vi "validate inputs.vi"(9 "output in":T3, 10 "process in":T1, 11 "input in":T2) -> (1 "output out":T3, 2 "process out":T1, 3 "input out":T2)   [LabVIEW 2013]
uses:
  Controls/output script control.ctl
  Controls/input script control.ctl
  Controls/processing script control.ctl
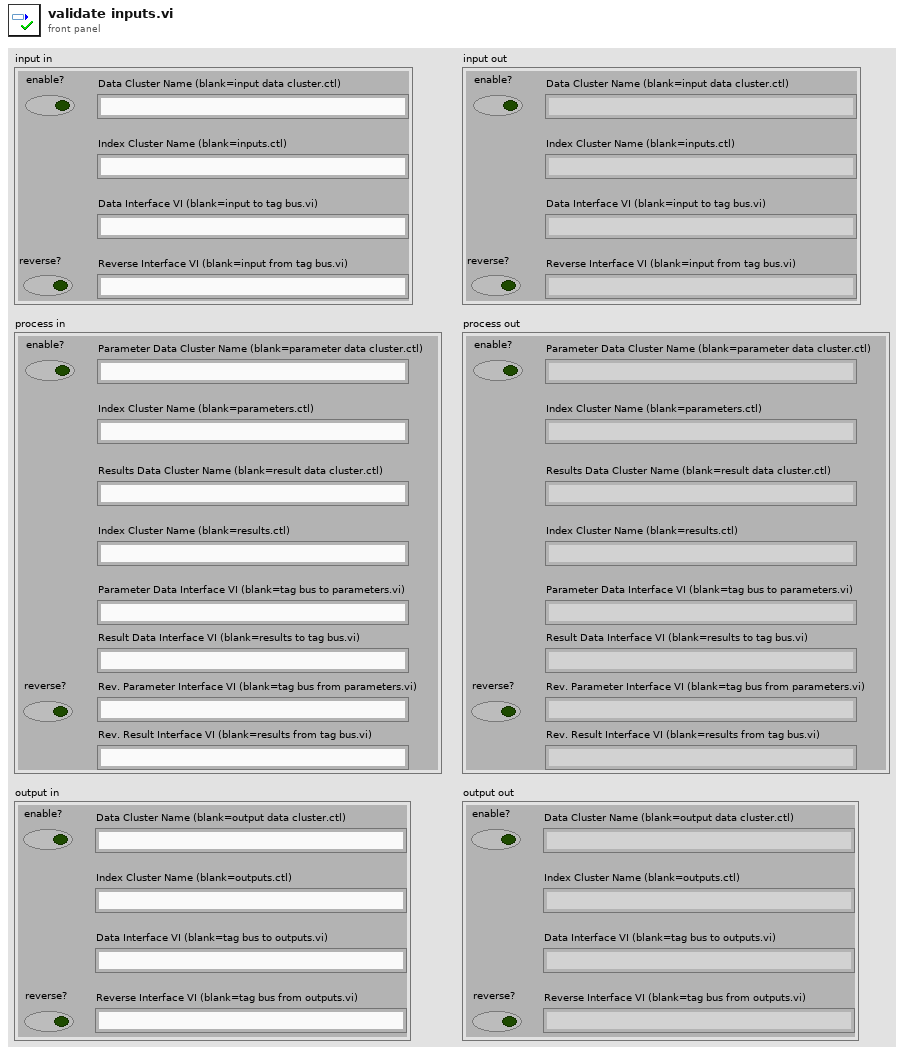
[diagram p1: front panel]
types:
  T1 = typedef "processing script control.ctl" = cluster{"enable?":bool, "Parameter Data Cluster Name (blank=parameter data cluster.ctl)":string, "Index Cluster Name (blank=parameters.ctl)":string, "Results Data Cluster Name (blank=result data cluster.ctl)":string, "Index Cluster Name (blank=results.ctl)":string, "Parameter Data Interface VI (blank=tag bus to parameters.vi)":string, "Result Data Interface VI (blank=results to tag bus.vi)":string, "reverse?":bool, "Rev. Result Interface VI (blank=results from tag bus.vi)":string, "Rev. Parameter Interface VI (blank=tag bus from parameters.vi)":string}
  T2 = typedef "input script control.ctl" = cluster{"enable?":bool, "Data Cluster Name (blank=input data cluster.ctl)":string, "Index Cluster Name (blank=inputs.ctl)":string, "Data Interface VI (blank=input to tag bus.vi)":string, "reverse?":bool, "Reverse Interface VI (blank=input from tag bus.vi)":string}
  T3 = typedef "output script control.ctl" = cluster{"enable?":bool, "Data Cluster Name (blank=output data cluster.ctl)":string, "Index Cluster Name (blank=outputs.ctl)":string, "Data Interface VI (blank=tag bus to outputs.vi)":string, "Reverse Interface VI (blank=tag bus from outputs.vi)":string, "reverse?":bool}
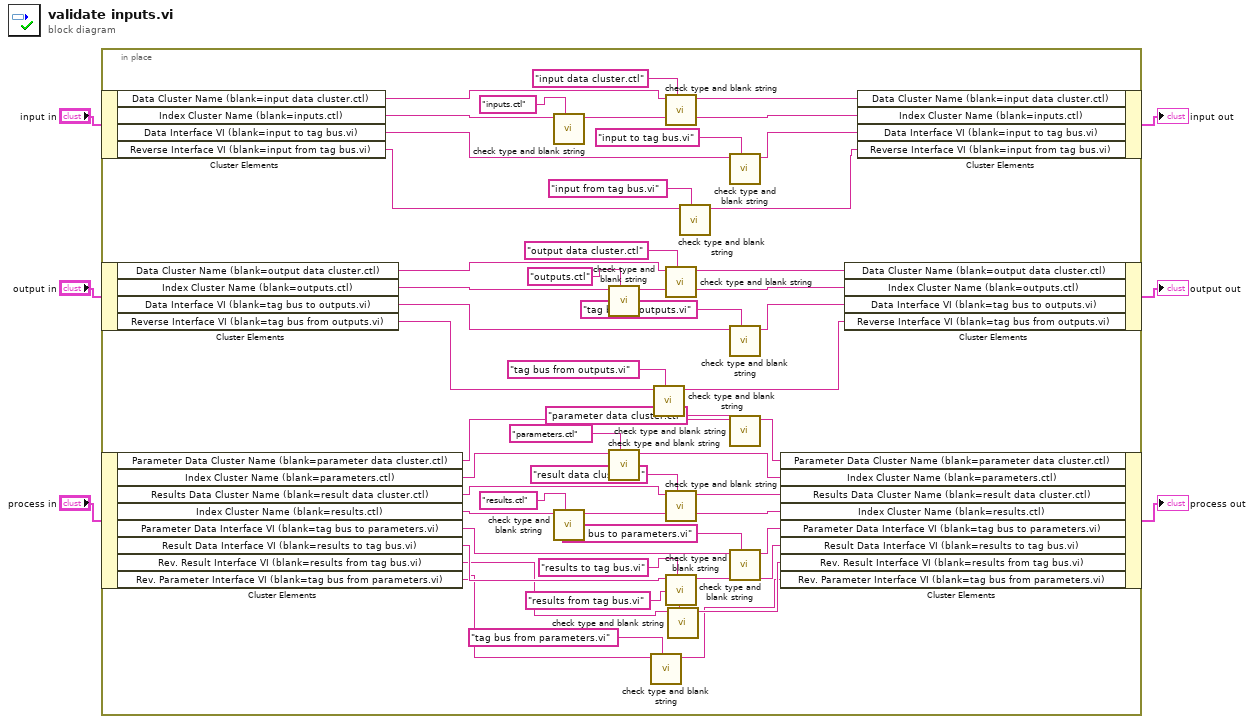
[diagram p0: block diagram]
diagram:
  n1 = in-place {
    n2 = in-place-cluster #1("input in") -> ("Data Cluster Name (blank=input data cluster.ctl)"=w53:string, "Index Cluster Name (blank=inputs.ctl)"=w51:string, "Data Interface VI (blank=input to tag bus.vi)"=w48:string, "Reverse Interface VI (blank=input from tag bus.vi)"=w16:string)
    n3 = in-place-cluster #2("output in") -> ("Data Cluster Name (blank=output data cluster.ctl)"=w42:string, "Index Cluster Name (blank=outputs.ctl)"=w47:string, "Data Interface VI (blank=tag bus to outputs.vi)"=w43:string, "Reverse Interface VI (blank=tag bus from outputs.vi)"=w14:string)
    n4 = in-place-cluster #3("process in") -> ("Parameter Data Cluster Name (blank=parameter data cluster.ctl)"=w35:string, "Index Cluster Name (blank=parameters.ctl)"=w34:string, "Results Data Cluster Name (blank=result data cluster.ctl)"=w33:string, "Index Cluster Name (blank=results.ctl)"=w32:string, "Parameter Data Interface VI (blank=tag bus to parameters.vi)"=w31:string, "Result Data Interface VI (blank=results to tag bus.vi)"=w30:string, "Rev. Result Interface VI (blank=results from tag bus.vi)"=w10:string, "Rev. Parameter Interface VI (blank=tag bus from parameters.vi)"=w7:string)
    n5 = call "check type and blank string.vi"("default"="inputs.ctl", "user input"=w51) -> ("validated"=w50:string)  [unwired: 9 in]
    n6 = call "check type and blank string.vi"("default"="results.ctl", "user input"=w32) -> ("validated"=w39:string)  [unwired: 9 in]
    n7 = call "check type and blank string.vi"("default"="outputs.ctl", "user input"=w47) -> ("validated"=w46:string)  [unwired: 9 in]
    n8 = call "check type and blank string.vi"("default"="parameters.ctl", "user input"=w34) -> ("validated"=w37:string)  [unwired: 9 in]
    n9 = call "check type and blank string.vi"("default"="tag bus from parameters.vi", "user input"=w7) -> ("validated"=w8:string)  [unwired: 9 in]
    n10 = call "check type and blank string.vi"("default"="tag bus from outputs.vi", "user input"=w14) -> ("validated"=w13:string)  [unwired: 9 in]
    n11 = call "check type and blank string.vi"("default"="input data cluster.ctl", "user input"=w53) -> ("validated"=w54:string)  [unwired: 9 in]
    n12 = call "check type and blank string.vi"("default"="output data cluster.ctl", "user input"=w42) -> ("validated"=w45:string)  [unwired: 9 in]
    n13 = call "check type and blank string.vi"("default"="result data cluster.ctl", "user input"=w33) -> ("validated"=w38:string)  [unwired: 9 in]
    n14 = call "check type and blank string.vi"("default"="results to tag bus.vi", "user input"=w30) -> ("validated"=w41:string)  [unwired: 9 in]
    n15 = call "check type and blank string.vi"("default"="results from tag bus.vi", "user input"=w10) -> ("validated"=w9:string)  [unwired: 9 in]
    n16 = call "check type and blank string.vi"("default"="input from tag bus.vi", "user input"=w16) -> ("validated"=w17:string)  [unwired: 9 in]
    n17 = call "check type and blank string.vi"("default"="input to tag bus.vi", "user input"=w48) -> ("validated"=w49:string)  [unwired: 9 in]
    n18 = call "check type and blank string.vi"("default"="tag bus to outputs.vi", "user input"=w43) -> ("validated"=w44:string)  [unwired: 9 in]
    n19 = call "check type and blank string.vi"("default"="parameter data cluster.ctl", "user input"=w35) -> ("validated"=w36:string)  [unwired: 9 in]
    n20 = call "check type and blank string.vi"("default"="tag bus to parameters.vi", "user input"=w31) -> ("validated"=w40:string)  [unwired: 9 in]
    n21 = in-place-cluster #3("Parameter Data Cluster Name (blank=parameter data cluster.ctl)"=w36, "Index Cluster Name (blank=parameters.ctl)"=w37, "Results Data Cluster Name (blank=result data cluster.ctl)"=w38, "Index Cluster Name (blank=results.ctl)"=w39, "Parameter Data Interface VI (blank=tag bus to parameters.vi)"=w40, "Result Data Interface VI (blank=results to tag bus.vi)"=w41, "Rev. Result Interface VI (blank=results from tag bus.vi)"=w9, "Rev. Parameter Interface VI (blank=tag bus from parameters.vi)"=w8) -> (→"process out":T1)
    n22 = in-place-cluster #2("Data Cluster Name (blank=output data cluster.ctl)"=w45, "Index Cluster Name (blank=outputs.ctl)"=w46, "Data Interface VI (blank=tag bus to outputs.vi)"=w44, "Reverse Interface VI (blank=tag bus from outputs.vi)"=w13) -> (→"output out":T3)
    n23 = in-place-cluster #1("Data Cluster Name (blank=input data cluster.ctl)"=w54, "Index Cluster Name (blank=inputs.ctl)"=w50, "Data Interface VI (blank=input to tag bus.vi)"=w49, "Reverse Interface VI (blank=input from tag bus.vi)"=w17) -> (→"input out":T2)
  }
